vi "practice 29.05.2025.vi"() -> ()   [LabVIEW 2021]
panel:
  in  "stop":bool
  out "Tab Control":enum32{"Page 1", "Page 2", "Page 3", "Page 4"}(tab)
  in  "1":bool
  in  "2":bool
  in  "3":bool
  in  "4":bool
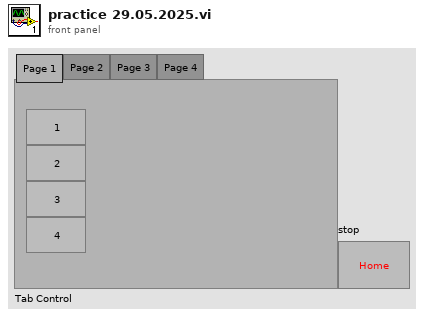
[diagram p1: front panel]
types:
  T1 = cluster{"Tab Control":enum32{"Page 1", "Page 2", "Page 3", "Page 4"}}
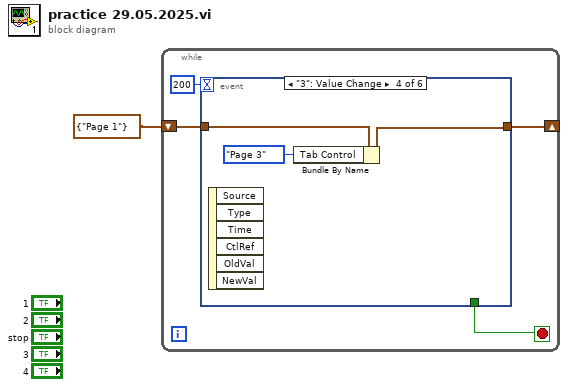
[diagram p0: block diagram]
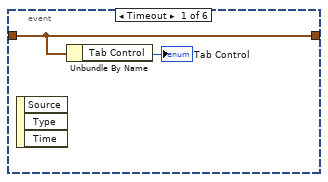
[diagram p2: hidden frame]
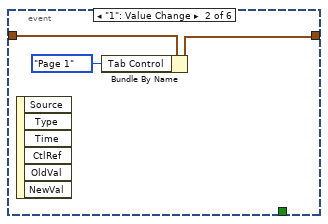
[diagram p3: hidden frame]
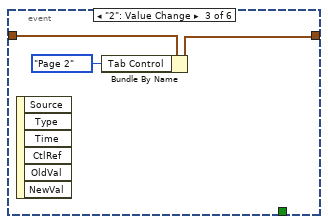
[diagram p4: hidden frame]
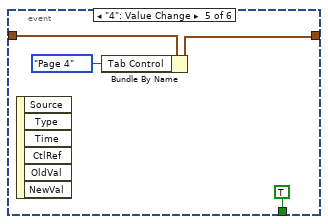
[diagram p5: hidden frame]
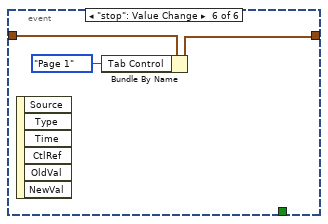
[diagram p6: hidden frame]
diagram:
  n1 = while {
    shift-right: [w4] -> _
    shift-left: T1 {"Tab Control"=enum."Page 1"} -> [w5]
    stop <- w3 stop-if-true
    n2 = event shown="[3] \"3\": Value Change" {
      selector: _ -> [_ _ _ _ _ _]
      dyn-events: _ -> [_ _ _ _ _ _]
      timeout: 200 -> [_ _ _ _ _ _]
      tunnel: w5 -> [w6 w10 w13 w16 w20 w23]
      tunnel: [w6 w9 w12 w15 w19 w22] -> w4
      tunnel: [_ _ _ _ TRUE _] -> w3
      event Timeout {
        n3 = event-data() -> ()  [unwired: 1 in, 3 out]
        n4 = Unbundle By Name(w6) -> ("Tab Control"=→"Tab Control":enum32{"Page 1", "Page 2", "Page 3", "Page 4"})
      }
      event "1": Value Change {
        n5 = event-data() -> ()  [unwired: 1 in, 6 out]
        n6 = Bundle By Name(cluster=w10, "Tab Control"=enum32{"Page 1", "Page 2", "Page 3", "Page 4"}."Page 1") -> (w9:T1)
      }
      event "2": Value Change {
        n7 = event-data() -> ()  [unwired: 1 in, 6 out]
        n8 = Bundle By Name(cluster=w13, "Tab Control"=enum32{"Page 1", "Page 2", "Page 3", "Page 4"}."Page 2") -> (w12:T1)
      }
      event "3": Value Change {
        n9 = event-data() -> ()  [unwired: 1 in, 6 out]
        n10 = Bundle By Name(cluster=w16, "Tab Control"=enum32{"Page 1", "Page 2", "Page 3", "Page 4"}."Page 3") -> (w15:T1)
      }
      event "4": Value Change {
        n11 = event-data() -> ()  [unwired: 1 in, 6 out]
        n12 = Bundle By Name(cluster=w20, "Tab Control"=enum32{"Page 1", "Page 2", "Page 3", "Page 4"}."Page 4") -> (w19:T1)
      }
      event "stop": Value Change {
        n13 = event-data() -> ()  [unwired: 1 in, 6 out]
        n14 = Bundle By Name(cluster=w23, "Tab Control"=enum32{"Page 1", "Page 2", "Page 3", "Page 4"}."Page 1") -> (w22:T1)
      }
    }
  }
